vi "Check and kill app.vi"(6 "Error Message in":string, 8 "Error In":errorcluster, 11 "Full App name (ex: PC Interface.exe)":string="PC Interface.exe") -> (0 "Error Out":errorcluster, 3 "app closed":bool, 4 "Error Message out":string)   [LabVIEW 2019]
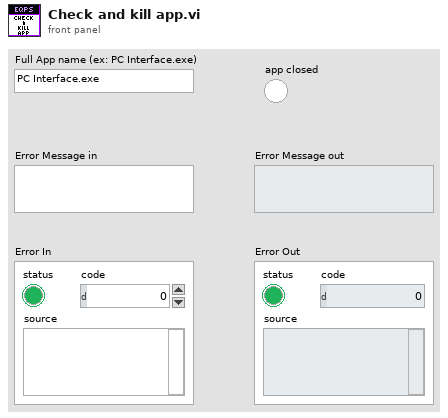
[diagram p1: front panel]
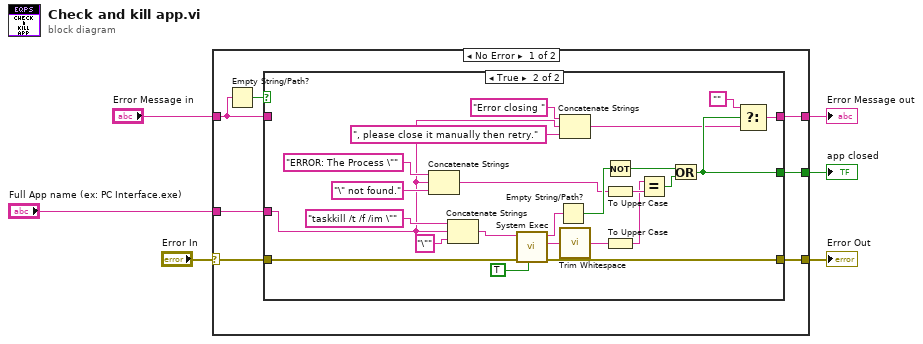
[diagram p0: block diagram]
diagram:
  n1 = case shown="No Error" "Error In" {
    selector: "Error In" -> [w9 w41]
    tunnel: [w10 w41] -> w5
    tunnel: [w12 w40] -> w4
    tunnel: "Error Message in" -> [w11 w40]
    tunnel: [w8 _] -> w2
    tunnel: "Full App name (ex: PC Interface.exe)" -> [w7 _]
    frame No Error {
      n2 = Empty String/Path?(string/path=w11) -> (empty?=w13:bool)
      n3 = case shown="True" w13 {
        tunnel: [w15 w30] -> w12
        tunnel: w11 -> [w15 _]
        tunnel: [w14 w38] -> w10
        tunnel: w9 -> [w14 w39]
        tunnel: [_ w32] -> w8
        tunnel: w7 -> [_ w19]
        frame False {
        }
        frame True {
          n4 = Concatenate Strings("ERROR: The Process \"", w19, "\" not found.") -> (w25:string)
          n5 = Concatenate Strings("taskkill /t /f /im \"", w19, "\"") -> (w18:string)
          n6 = call <vilib>:"System Exec.vi"("run minimized? (F)"=TRUE, "error in (no error)"=w39, "command line"=w18) -> ("error out"=w38:errorcluster, "standard error"=w37:string, "standard output"=w36:string)  [unwired: 5 in, 1 out]
          n7 = Empty String/Path?(string/path=w36) -> (empty?=w35:bool)
          n8 = Concatenate Strings("Error closing ", w19, ", please close it manually then retry.") -> (w22:string)
          n9 = call <vilib>:"Trim Whitespace.vi"("string"=w37) -> ("trimmed string"=w29:string)  [unwired: 1 in]
          n10 = Not(x=w35) -> (.not. x?=w33:bool)
          n11 = To Upper Case(1:w25) -> (0:w17:string)
          n12 = To Upper Case(1:w29) -> (0:w16:string)
          n13 = Equal?(x=w16, y=w17) -> (x = y?=w34:bool)
          n14 = Or(x=w33, y=w34) -> (x .or. y?=w32:bool)
          n15 = Select(t="", s=w32, f=w22) -> (s? t:f=w30:string)
        }
      }
    }
    frame Error {
    }
  }
  "Error Out" <- w5
  "Error Message out" <- w4
  "app closed" <- w2
